vi "Generate Unique Header.vi"(8 "error in":errorcluster, 11 "Vaisala Data in":refnum<class "Vaisala Data.lvclass">) -> (0 "error out":errorcluster, 2 "Header":string[](array[string]), 3 "Vaisala Data out":refnum<class "Vaisala Data.lvclass">)   [LabVIEW 2015, in "Vaisala Library.lvlib" / "Vaisala Data.lvclass"]
uses:
  Vaisala Data.lvclass
  <vilib>/MSR Consulting, LLC/General Reuse/Data/Data.lvclass/Data.ctl
  <vilib>/MSR Consulting, LLC/General Reuse/Data/Read Data ID.vi
  <vilib>/MSR Consulting, LLC/General Reuse/Data/Data.lvclass
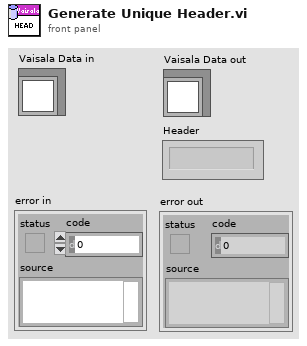
[diagram p1: front panel]
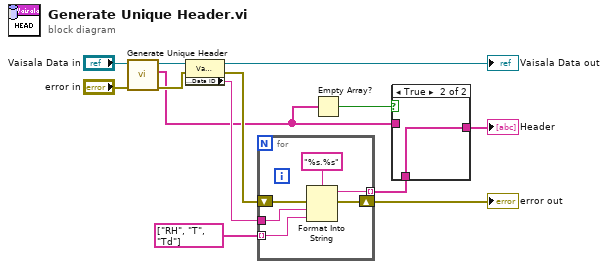
[diagram p0: block diagram]
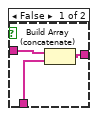
[diagram p2: hidden frame]
diagram:
  n1 = call-parent "Generate Unique Header.vi"("error in"="error in", "Data in"="Vaisala Data in") -> ("error out"=w9:errorcluster, "Header"=w2:string[], "Data out"=w11:refnum<class "Vaisala Data.lvclass">)  [unwired: 7 in]
  n2 = property class="Vaisala Data"(reference=w11, error in=w9) -> (reference out=→"Vaisala Data out":refnum<class "Vaisala Data.lvclass">, error out=w6:errorcluster, "Accessors:Data ID"=w8:string)
  n3 = for {
    tunnel: w8 -> [w19]
    tunnel: [w17] -> w4 mode=indexing
    tunnel: string[] ["RH", "T", "Td"] -> [w16] mode=indexing
    shift-right: [w15] -> w5
    shift-left: w6 -> [w14]
    n4 = Format Into String(format string="%s.%s", error in=w14, w19, w16) -> (resulting string=w17:string, error out=w15:errorcluster)  [unwired: 1 in]
  }
  "error out" <- w5
  n5 = Empty Array?(array=w2) -> (empty?=w1:bool)
  n6 = case shown="True" w1 {
    tunnel: w4 -> [w22 w23]
    tunnel: [w21 w23] -> w3
    tunnel: w2 -> [w20 _]
    frame False {
      n7 = Build Array (concatenate)(w20, w22) -> (w21:string[])
    }
    frame True {
    }
  }
  "Header" <- w3
